vi "Helmholtz2D_Cal RHS_Update BC.vi"(8 "Domain":T2={"x"={"start x"=0.0, "end x"=1.0, "# of x-points"=11}, "y"={"start y"=0.0, "end y"=1.0, "# of y-points"=11}}, 9 "k":dbl=1.0, 10 "F(x, y)":dbl[][](array[numeric]), 11 "Boundary Condition In":cluster{"type":T1, "Value":dbl[]}[](array[cluster]) {"type" items=["Dirichlet", "Neumann"]}) -> (3 "Boundary Condition Out":cluster{"type":T1, "Value":dbl[]}[](array[cluster]) {"type" items=["Dirichlet", "Neumann"]})   [LabVIEW 2020, in "NI_PDE.lvlib"]
uses:
  <vilib>/gmath/NI_PDE.lvlib
  <vilib>/gmath/pde.llb/Common/PDE_BC Type.ctl
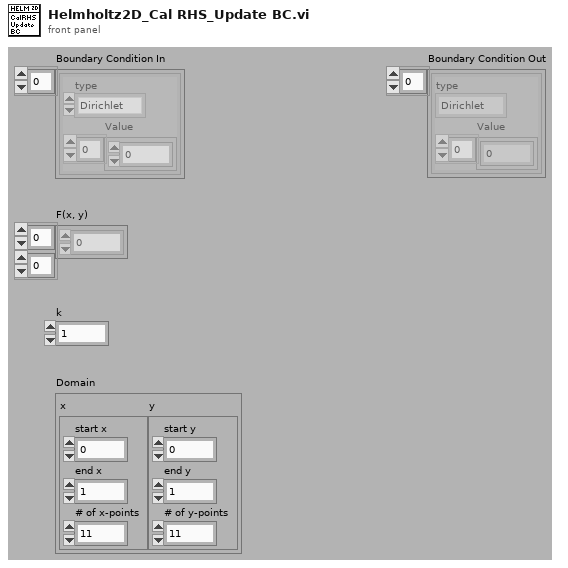
[diagram p1: front panel]
types:
  T1 = typedef "NI_PDE.lvlib/PDE_BC Type.ctl" = i32
  T2 = cluster{"x":cluster{"start x":dbl, "end x":dbl, "# of x-points":i32}, "y":cluster{"start y":dbl, "end y":dbl, "# of y-points":i32}}
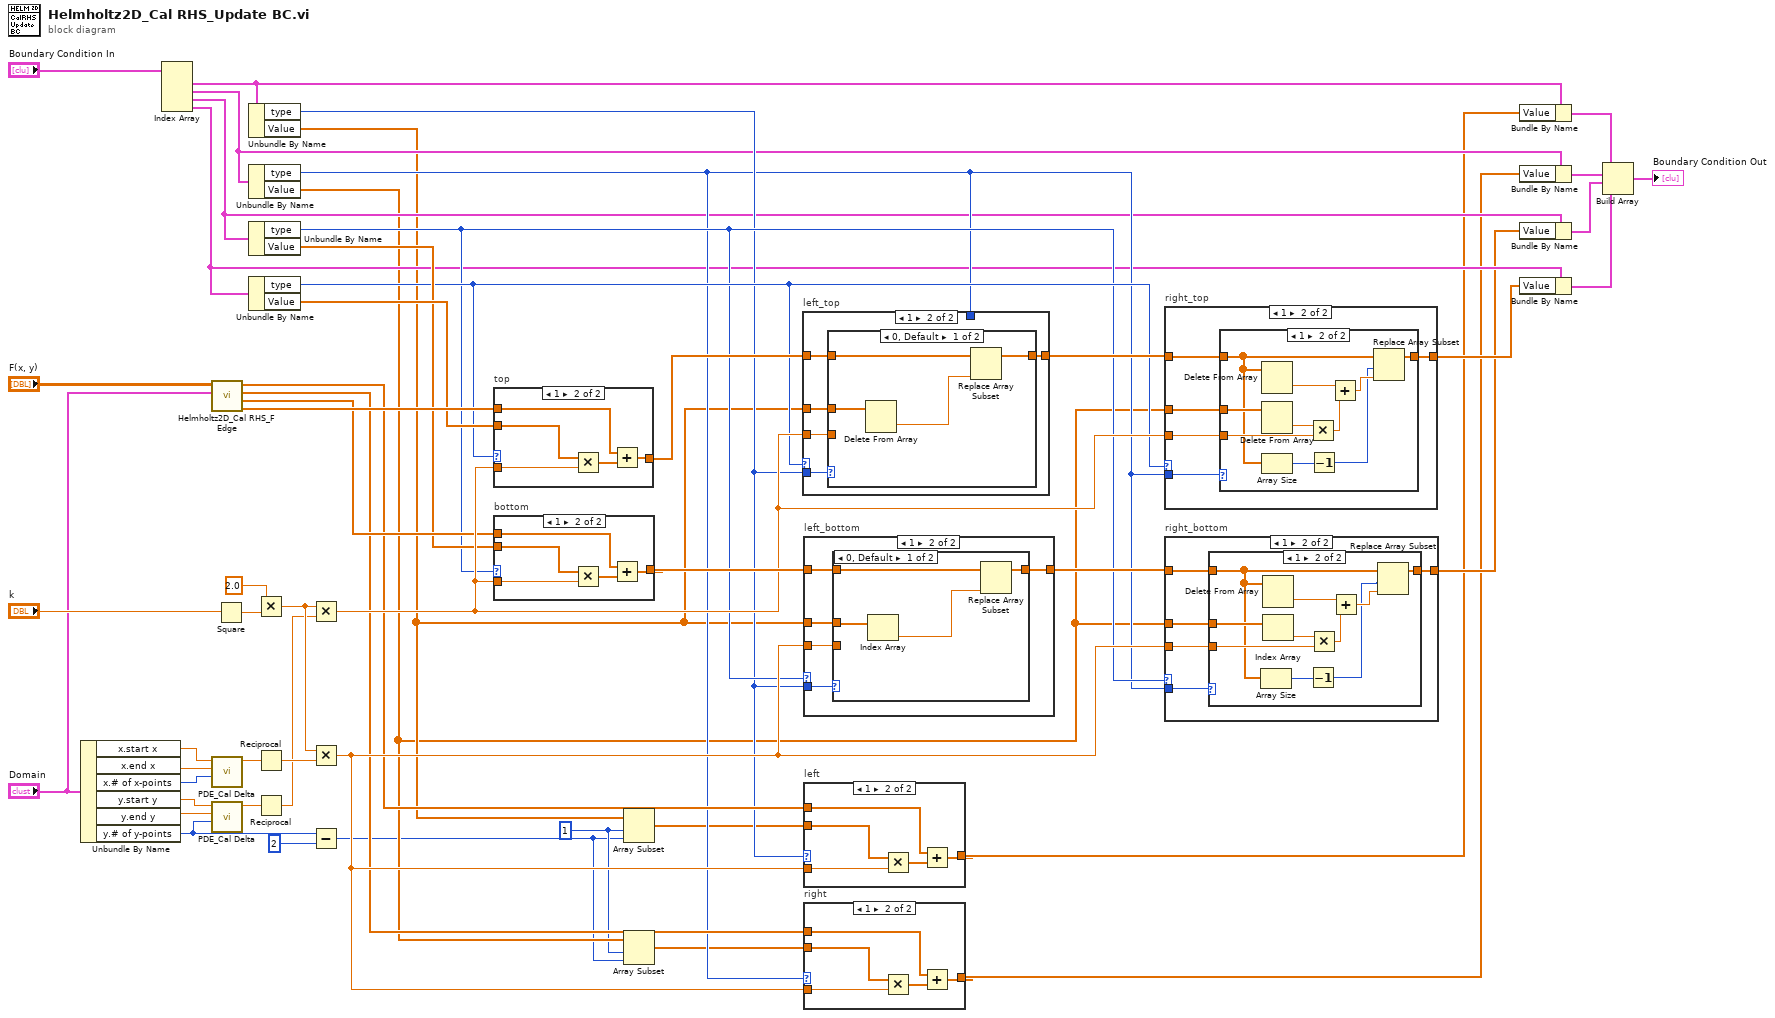
[diagram p0: block diagram]
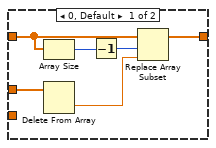
[diagram p3: hidden frame]
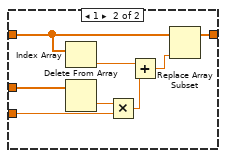
[diagram p5: hidden frame]
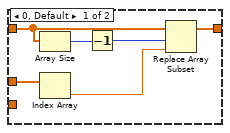
[diagram p7: hidden frame]
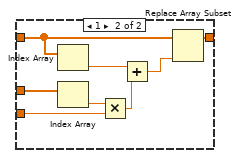
[diagram p13: hidden frame]
diagram:
  w4 = 1 ("index")
  n1 = Unbundle By Name("Domain") -> ("x.start x"=w53:dbl, "x.end x"=w52:dbl, "x.# of x-points"=w49:i32, "y.start y"=w50:dbl, "y.end y"=w51:dbl, "y.# of y-points"=w9:i32)
  n2 = Index Array(array="Boundary Condition In") -> (element #1=w16:cluster{"type":T1, "Value":dbl[]}, element #2=w18:cluster{"type":T1, "Value":dbl[]}, element #3=w20:cluster{"type":T1, "Value":dbl[]}, element #4=w23:cluster{"type":T1, "Value":dbl[]})  [unwired: 4 in]
  n3 = call <vilib>:"Helmholtz2D_Cal RHS_F Edge.vi"("Domain"="Domain", "F(x, y)"="F(x, y)") -> ("F End Y"=w33:dbl[], "F Start Y"=w32:dbl[], "F End X"=w30:dbl[], "F Start X"=w31:dbl[])  [unwired: 6 out]
  n4 = call <vilib>:"PDE_Cal Delta.vi"("# of points"=w49, "end"=w52, "start"=w53) -> ("delta"=w38:dbl)  [unwired: 8 out]
  n5 = call <vilib>:"PDE_Cal Delta.vi"("# of points"=w9, "end"=w51, "start"=w50) -> ("delta"=w37:dbl)  [unwired: 8 out]
  n6 = Square(x="k") -> (x^2=w47:dbl)
  n7 = Unbundle By Name(w16) -> ("type"=w25:T1, "Value"=w7:dbl[])
  n8 = Unbundle By Name(w18) -> ("type"=w24:T1, "Value"=w5:dbl[])
  n9 = Unbundle By Name(w20) -> ("type"=w26:T1, "Value"=w28:dbl[])
  n10 = Unbundle By Name(w23) -> ("type"=w27:T1, "Value"=w29:dbl[])
  n11 = Multiply(x=2.0, y=w47) -> (x*y=w46:dbl)
  n12 = Reciprocal(x=w38) -> (1/x=w2:dbl)
  n13 = Reciprocal(x=w37) -> (1/x=w1:dbl)
  n14 = Multiply(x=w46, y=w1) -> (x*y=w40:dbl)
  n15 = Multiply(x=w46, y=w2) -> (x*y=w43:dbl)
  n16 = Subtract(x=w9, y=2) -> (x-y=w3:i32)
  n17 = case "top" shown="1" w27 {
    tunnel: w29 -> [w54 w55]
    tunnel: w40 -> [_ w59]
    tunnel: [w54 w57] -> w41
    tunnel: w33 -> [_ w56]
    frame 0, Default {
    }
    frame 1 {
      n18 = Multiply(x=w55, y=w59) -> (x*y=w58:dbl[])
      n19 = Add(x=w56, y=w58) -> (x+y=w57:dbl[])
    }
  }
  n20 = case "bottom" shown="1" w26 {
    tunnel: w28 -> [w60 w61]
    tunnel: w40 -> [_ w65]
    tunnel: [w60 w63] -> w45
    tunnel: w32 -> [_ w62]
    frame 0, Default {
    }
    frame 1 {
      n21 = Multiply(x=w61, y=w65) -> (x*y=w64:dbl[])
      n22 = Add(x=w62, y=w64) -> (x+y=w63:dbl[])
    }
  }
  n23 = Array Subset(array=w7, index=w4, length=w3) -> (w10:dbl[])
  n24 = Array Subset(array=w5, index=w4, length=w3) -> (w6:dbl[])
  n25 = case "left_top" shown="1" w27 {
    tunnel: w41 -> [w66 w70]
    tunnel: [w66 w71] -> w42
    tunnel: w7 -> [_ w69]
    tunnel: w40 -> [_ w68]
    tunnel: w25 -> [_ w67]
    tunnel: w24 -> [_ _]
    frame 0, Default {
    }
    frame 1 {
      n26 = case shown="0, Default" w67 {
        tunnel: [w73 w83] -> w71
        tunnel: w70 -> [w74 w81]
        tunnel: w69 -> [w75 w80]
        tunnel: w68 -> [_ w77]
        frame 0, Default {
          n27 = Delete From Array(array=w75) -> (deleted portion=w72:dbl)  [unwired: 2 in, 1 out]
          n28 = Replace Array Subset(array=w74, new element=w72) -> (w73:dbl[])  [unwired: 1 in]
        }
        frame 1 {
          n29 = Index Array(array=w81) -> (element=w82:dbl)  [unwired: 1 in]
          n30 = Delete From Array(array=w80) -> (deleted portion=w78:dbl)  [unwired: 2 in, 1 out]
          n31 = Multiply(x=w78, y=w77) -> (x*y=w76:dbl)
          n32 = Add(x=w82, y=w76) -> (x+y=w79:dbl)
          n33 = Replace Array Subset(array=w81, new element=w79) -> (w83:dbl[])  [unwired: 1 in]
        }
      }
    }
  }
  n34 = case "left_bottom" shown="1" w26 {
    tunnel: w45 -> [w84 w88]
    tunnel: [w84 w89] -> w44
    tunnel: w7 -> [_ w87]
    tunnel: w43 -> [_ w86]
    tunnel: w25 -> [_ w85]
    frame 0, Default {
    }
    frame 1 {
      n35 = case shown="0, Default" w85 {
        tunnel: [w91 w101] -> w89
        tunnel: w88 -> [w92 w99]
        tunnel: w87 -> [w93 w98]
        tunnel: w86 -> [_ w95]
        frame 0, Default {
          n36 = Index Array(array=w93) -> (element=w90:dbl)  [unwired: 1 in]
          n37 = Replace Array Subset(array=w92, new element=w90) -> (w91:dbl[])  [unwired: 1 in]
        }
        frame 1 {
          n38 = Index Array(array=w99) -> (element=w100:dbl)  [unwired: 1 in]
          n39 = Index Array(array=w98) -> (element=w96:dbl)  [unwired: 1 in]
          n40 = Multiply(x=w96, y=w95) -> (x*y=w94:dbl)
          n41 = Add(x=w100, y=w94) -> (x+y=w97:dbl)
          n42 = Replace Array Subset(array=w99, new element=w97) -> (w101:dbl[])  [unwired: 1 in]
        }
      }
    }
  }
  n43 = case "left" shown="1" w25 {
    tunnel: w10 -> [w102 w103]
    tunnel: w43 -> [_ w107]
    tunnel: [w102 w105] -> w17
    tunnel: w31 -> [_ w104]
    frame 0, Default {
    }
    frame 1 {
      n44 = Multiply(x=w103, y=w107) -> (x*y=w106:dbl[])
      n45 = Add(x=w104, y=w106) -> (x+y=w105:dbl[])
    }
  }
  n46 = case "right" shown="1" w24 {
    tunnel: w6 -> [w108 w109]
    tunnel: w43 -> [_ w113]
    tunnel: [w108 w111] -> w19
    tunnel: w30 -> [_ w110]
    frame 0, Default {
    }
    frame 1 {
      n47 = Multiply(x=w109, y=w113) -> (x*y=w112:dbl[])
      n48 = Add(x=w110, y=w112) -> (x+y=w111:dbl[])
    }
  }
  n49 = case "right_top" shown="1" w27 {
    tunnel: w42 -> [w114 w118]
    tunnel: [w114 w119] -> w22
    tunnel: w5 -> [_ w117]
    tunnel: w40 -> [_ w116]
    tunnel: w24 -> [_ w115]
    frame 0, Default {
    }
    frame 1 {
      n50 = case shown="1" w115 {
        tunnel: [w123 w135] -> w119
        tunnel: w118 -> [w121 w127]
        tunnel: w117 -> [w125 w133]
        tunnel: w116 -> [_ w130]
        frame 0, Default {
          n51 = Array Size(array=w121) -> (size(s)=w122:i32)
          n52 = Delete From Array(array=w125) -> (deleted portion=w124:dbl)  [unwired: 2 in, 1 out]
          n53 = Decrement(x=w122) -> (x-1=w120:i32)
          n54 = Replace Array Subset(array=w121, new element=w124, index=w120) -> (w123:dbl[])
        }
        frame 1 {
          n55 = Delete From Array(array=w127) -> (deleted portion=w134:dbl)  [unwired: 2 in, 1 out]
          n56 = Delete From Array(array=w133) -> (deleted portion=w131:dbl)  [unwired: 2 in, 1 out]
          n57 = Array Size(array=w127) -> (size(s)=w128:i32)
          n58 = Multiply(x=w131, y=w130) -> (x*y=w129:dbl)
          n59 = Decrement(x=w128) -> (x-1=w126:i32)
          n60 = Add(x=w134, y=w129) -> (x+y=w132:dbl)
          n61 = Replace Array Subset(array=w127, new element=w132, index=w126) -> (w135:dbl[])
        }
      }
    }
  }
  n62 = case "right_bottom" shown="1" w26 {
    tunnel: w44 -> [w136 w140]
    tunnel: [w136 w141] -> w21
    tunnel: w5 -> [_ w139]
    tunnel: w43 -> [_ w138]
    tunnel: w24 -> [_ w137]
    frame 0, Default {
    }
    frame 1 {
      n63 = case shown="1" w137 {
        tunnel: [w146 w157] -> w141
        tunnel: w140 -> [w144 w149]
        tunnel: w139 -> [w147 w155]
        tunnel: w138 -> [_ w152]
        frame 0, Default {
          n64 = Array Size(array=w144) -> (size(s)=w143:i32)
          n65 = Index Array(array=w147) -> (element=w145:dbl)  [unwired: 1 in]
          n66 = Decrement(x=w143) -> (x-1=w142:i32)
          n67 = Replace Array Subset(array=w144, new element=w145, index=w142) -> (w146:dbl[])
        }
        frame 1 {
          n68 = Array Size(array=w149) -> (size(s)=w150:i32)
          n69 = Delete From Array(array=w149) -> (deleted portion=w156:dbl)  [unwired: 2 in, 1 out]
          n70 = Index Array(array=w155) -> (element=w153:dbl)  [unwired: 1 in]
          n71 = Decrement(x=w150) -> (x-1=w148:i32)
          n72 = Multiply(x=w153, y=w152) -> (x*y=w151:dbl)
          n73 = Add(x=w156, y=w151) -> (x+y=w154:dbl)
          n74 = Replace Array Subset(array=w149, new element=w154, index=w148) -> (w157:dbl[])
        }
      }
    }
  }
  n75 = Bundle By Name(cluster=w16, "Value"=w17) -> (w15:cluster{"type":T1, "Value":dbl[]})
  n76 = Bundle By Name(cluster=w18, "Value"=w19) -> (w14:cluster{"type":T1, "Value":dbl[]})
  n77 = Bundle By Name(cluster=w20, "Value"=w21) -> (w13:cluster{"type":T1, "Value":dbl[]})
  n78 = Bundle By Name(cluster=w23, "Value"=w22) -> (w12:cluster{"type":T1, "Value":dbl[]})
  n79 = Build Array(w15, w14, w13, w12) -> (→"Boundary Condition Out":cluster{"type":T1, "Value":dbl[]}[])
